vi "data_test.vi"() -> ()   [LabVIEW 2017]
uses:
  <vilib>/addons/database/Connection.llb/DB Tools Open Connec (Path).vi
  <vilib>/addons/database/NI_Database_API.lvlib
panel:
  in  "current time":timestamp
  out "output cluster":cluster{"available":string, dbl}
  out "error out 2":errorcluster
  out "error out":errorcluster
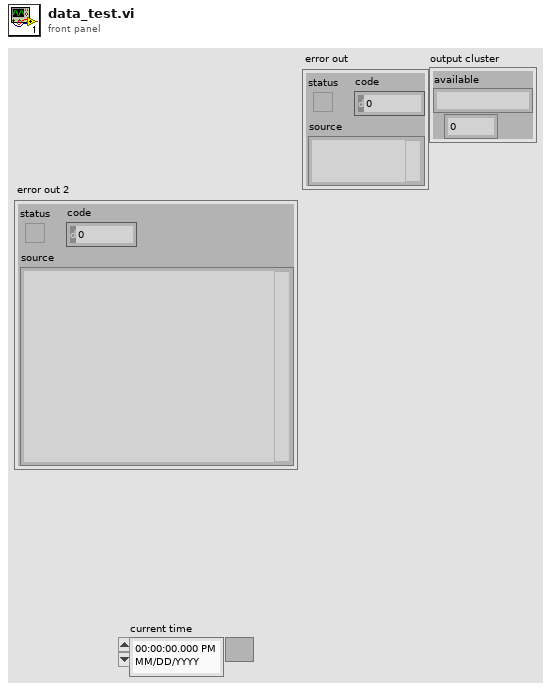
[diagram p1: front panel]
types:
  T1 = typedef "NI_Database_API.lvlib/Conn ObjectReference.ctl" = refnum<k1>
  T2 = cluster{"seconds since 1Jan1904":timestamp, "available":string, dbl}
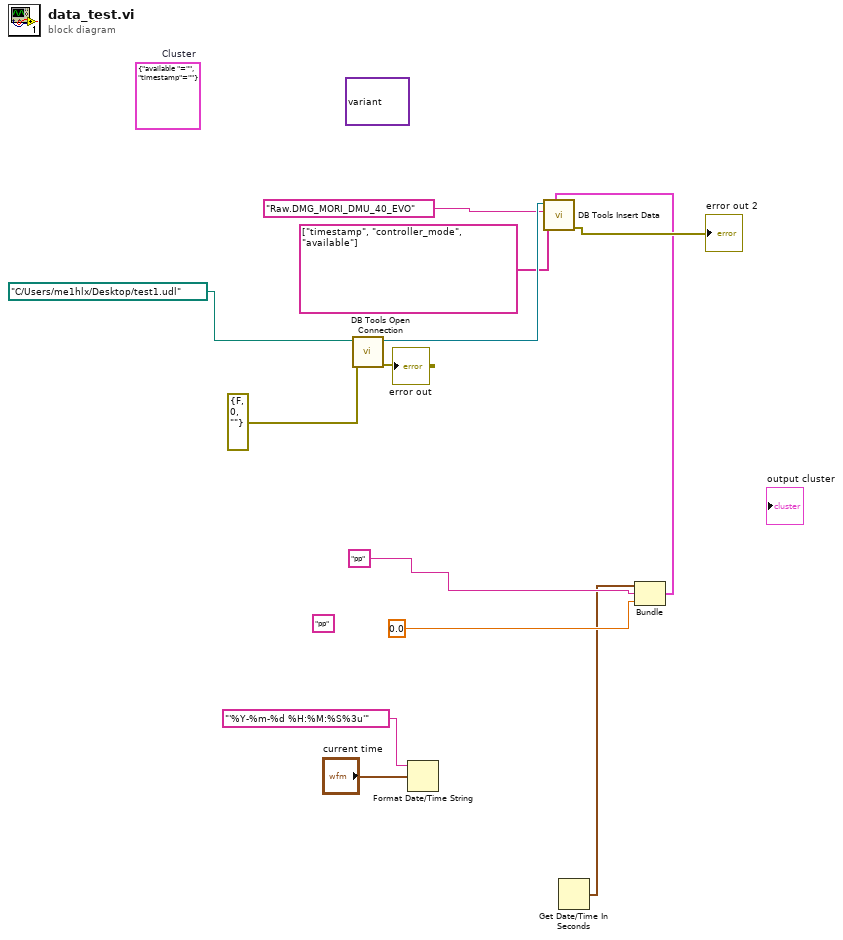
[diagram p0: block diagram]
diagram:
  (unwired) "pp" ("available")
  (unwired) variant(cluster{string, string} {"hhh", "pp"}) ("data")
  (unwired) cluster{"available ":string, "timestamp":string} {"available "="", "timestamp"=""}  # Cluster
  n1 = call-poly <vilib>:"DB Tools Open Connection.vi"("error in (no error)"=errorcluster {"status"=FALSE, "code"=0, "source"=""}, "connection information"=path "C:/Users/me1hlx/Desktop/test1.udl") -> ("error out"=→"error out":errorcluster, "connection reference"=w10:T1)  [unwired: 6 in]
  n2 = Format Date/Time String(time format string (%c)="'%Y-%m-%d %H:%M:%S%3u'", seconds (now)="current time") -> ()  [unwired: 1 in, 1 out]
  n3 = Get Date/Time In Seconds() -> (seconds since 1Jan1904=w1:timestamp)
  n4 = Bundle("seconds since 1Jan1904"=w1, "available"="pp", 0.0) -> (w4:T2)  [unwired: 1 in]
  n5 = call <vilib>:"DB Tools Insert Data.vi"("data"=w4, "columns"=string[] ["timestamp", "controller_mode", "available"], "table"="Raw.DMG_MORI_DMU_40_EVO", "connection reference"=w10) -> ("error out"=→"error out 2":errorcluster)  [unwired: 6 in, 1 out]
